vi "PH_Cam_BaseClass.constructor.vi"(0 "name":string, 2 "data in":string, 5 "error in(no error)":errorcluster) -> (14 "i ref out":refnum<vi>, 16 "data out":string, 19 "error out":errorcluster)   [LabVIEW 2014, in "PH_Cam_BaseClass.lvlib"]
doc: "This class controls a IEEE 1394 camera.\n\nThis class is part of the PHELIX user layer.\n\nauthor: Stefan Götte, GSI\n\nLicense Agreement for this software:\n\nCopyright (C)\nGesellschaft für Schwerionenforschung, GSI\nPlanckstr. 1\n64291 Darmstadt\nGermany\n\nContact: D.Beck@gsi.de \n\nThis program is free software; you can redistribute it and/or modify it under the terms of the \nGNU General Public License as published by the Free Software Foundation; either version 2 of \nthe license, or (at your option) any later version.\n\nThis program is distributed in the hope that it will be useful, but WITHOUT ANY WARRANTY; \nwithout even the implied warranty of MERCHANTABILITY or FITNESS FOR A PARTICULAR PURPOSE. See the GNU General License for more details (http://www.gnu.org).\n\nGesellschaft für Schwerionenforschung, GSI\nPlanckstr. 1, 64291 Darmstadt, Germany\nFor all questions and ideas contact: M.Richter@gsi.de, H.Brand@gsi.de or D.Beck@gsi.de.\nLast update: 16-JUN-2004"
uses:
  PH_Cam_BaseClass.lvlib
  PH_PSDBWriter/PH_PSDBWriter.lvlib
  CSCore/CSSystem/CSSystemLib/CSSystemLib.lvlib
  PH_Class/PH_Class.lvlib
  PH_StatusHandler/PH_StatusHandler.lvlib
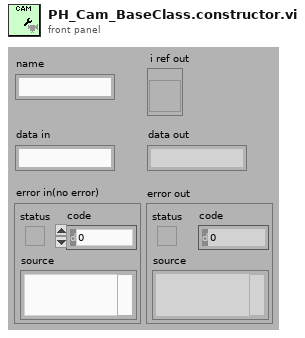
[diagram p1: front panel]
types:
  T1 = enum16{"SetAttribute", "GetAttribute", "CreateAttribute", "DestroyAttribute", "DestroyAllAtributes"}
  T2 = typedef "PH_Cam_BaseClass.lvlib/PH_Cam_BaseClass.Image Type.ctl" = cluster{"Set?":bool, "Image Type":T3}
  T3 = typedef "Image Type" = u32
  T4 = typedef "PH_Cam_BaseClass.lvlib/PH_Cam_BaseClass.i attribute.ctl" = cluster{"Gui Refs":T5, "Cam":cluster{"Source Notifier":refnum<notifier>, "Error":errorcluster, "Camera ID":string}, "Images":cluster{"Cam":T6, "Operation":T6, "PSDB":T6}, "Window Image":cluster{"Indicate Image":bool, "Window No.":i32, "Scale Facor":dbl, "Center Cross":bool, "Subtract Backgr":bool, "CoG":bool, "Color Palette":cluster{"Red":u8, "Green":u8, "Blue":u8}[], "Image On":bool}, "Default Prdc Int":i32, "Performance":cluster{"on":bool, "Timestamp Last Frame":i32}, "Histogram":cluster{"on":bool, "Mapping":bool}, "Save Image":cluster{"Save":bool, "File refnum":refnum<file>}, "Setting Service ID":i32, "Screen":cluster{"x-resolution":i16, "y-resolution":i16}, "On":bool, "Constructor finished":bool, "configured":bool}
  T5 = typedef "PH_Cam_BaseClass.lvlib/PH_Cam_BaseClass.GUI Refs.ctl" = cluster{"Frame Rate":refnum<vi>, "Get Frame Rate":refnum<vi>, "Show Image":refnum<vi>, "Get Histogram":refnum<vi>, "Mapping":refnum<vi>, "Histogram":refnum<vi>, "Center Cross":refnum<vi>, "Center of Gravity":refnum<vi>, "Scale Factor [%]":refnum<vi>, "Save Image":refnum<vi>, "Palette":refnum<vi>, "Subtract Background":refnum<vi>, "Cam Error":refnum<vi>, "On":refnum<vi>, "Cam List":refnum<vi>}
  T6 = typedef "IMAQ Image.ctl" = refnum<image>
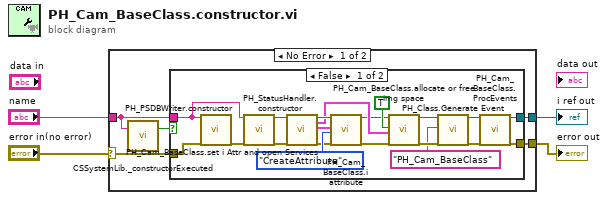
[diagram p0: block diagram]
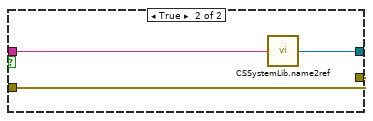
[diagram p2: hidden frame]
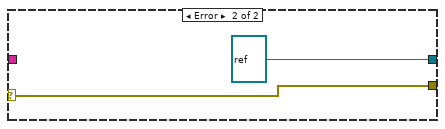
[diagram p3: hidden frame]
diagram:
  n1 = case shown="No Error" "error in(no error)" {
    selector: "error in(no error)" -> [w9 w34]
    tunnel: [w8 refnum<vi> refnum ("i ref out")] -> w4
    tunnel: [w7 w34] -> w3
    tunnel: "name" -> [w6 _]
    frame No Error {
      n2 = call "CSSystemLib._constructorExecuted.vi"("name"=w6) -> ("constructor executed?"=w5:bool)  [unwired: 18 in]
      n3 = case shown="False" w5 {
        tunnel: w9 -> [w16 w32]
        tunnel: [w27 w30] -> w8
        tunnel: [w26 w32] -> w7
        tunnel: w6 -> [w10 w31]
        frame False {
          n4 = call "PH_PSDBWriter.constructor.vi"("name"=w10, "error in"=w16) -> ("error out"=w22:errorcluster)  [unwired: 15 in, 2 out]
          n5 = call "PH_StatusHandler.constructor.vi"("name"=w10, "error in(no error)"=w22) -> ("i ref out"=w11:refnum<vi>, "error out"=w12:errorcluster)  [unwired: 15 in, 1 out]
          n6 = call "PH_Cam_BaseClass.set i Attr and open Services.vi"("i ref in"=w11, "error in (no error)"=w12) -> ("i ref out"=w24:refnum<vi>, "Image Type"=w15:T2, "i Attributes"=w23:T4, "error out"=w25:errorcluster)  [unwired: 14 in]
          n7 = call "PH_Cam_BaseClass.i attribute.vi"("VI Refnum"=w24, "CLASS.i attribute"=w23, "Action"=T1."CreateAttribute", "error in (no error)"=w25) -> ("VI Refnum out"=w13:refnum<vi>, "error out"=w14:errorcluster)  [unwired: 13 in, 1 out]
          n8 = call "PH_Cam_BaseClass.allocate or free img space.vi"("i ref in"=w13, "Allocate?"=TRUE, "Image Type"=w15, "error in (no error)"=w14) -> ("i ref out"=w21:refnum<vi>, "error out"=w20:errorcluster)  [unwired: 14 in]
          n9 = call "PH_Class.Generate Event.vi"("i ref in"=w21, "Class"="PH_Cam_BaseClass", "error in (no error)"=w20) -> ("i ref out"=w19:refnum<vi>, "error out"=w18:errorcluster)  [unwired: 15 in]
          n10 = call "PH_Cam_BaseClass.ProcEvents.vi"("i ref in"=w19, "error in"=w18) -> ("i ref out"=w27:refnum<vi>, "error out"=w26:errorcluster)  [unwired: 16 in]
        }
        frame True {
          n11 = call "CSSystemLib.name2ref.vi"("name"=w31) -> ("obj refnum"=w30:refnum<vi>)
        }
      }
    }
    frame Error {
    }
  }
  "i ref out" <- w4
  "error out" <- w3
